vi "Read Current Position.vi"(8 "error in":errorcluster, 11 "Axis in":refnum<class "Axis.lvclass">) -> (0 "error out":errorcluster, 2 "Current Position":dbl, 3 "Axis out":refnum<class "Axis.lvclass">)   [LabVIEW 2018, in "Axis.lvlib" / "Axis.lvclass"]
uses:
  Axis.lvclass
  Axis.lvclass/Axis.ctl
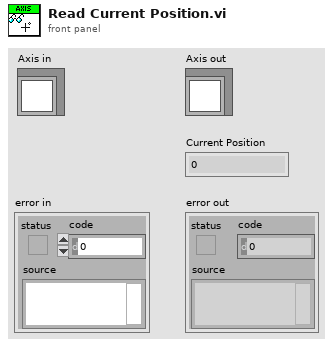
[diagram p1: front panel]
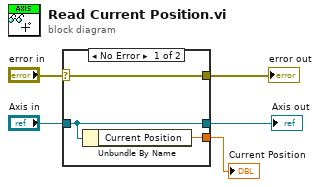
[diagram p0: block diagram]
diagram:
  n1 = case shown="No Error" "error in" {
    selector: "error in" -> [w8 w9]
    tunnel: [w8 w9] -> w4
    tunnel: [w7 w10] -> w2
    tunnel: "Axis in" -> [w7 w10]
    tunnel: [w6 _] -> w1
    frame No Error {
      n2 = Unbundle By Name(w7) -> ("Current Position"=w6:dbl)
    }
    frame Error {
    }
  }
  "error out" <- w4
  "Axis out" <- w2
  "Current Position" <- w1
